vi "Parse JSON detailed err.vi"(8 "error in (no error)":errorcluster, 11 "JSON string in":string) -> (0 "error out":errorcluster, 3 "long err description out":string)   [LabVIEW 2018, in "LabView-0mq-Jl_Roundtrip_lib.lvlib"]
uses:
  LabView-0mq-Jl_Roundtrip_lib.lvlib
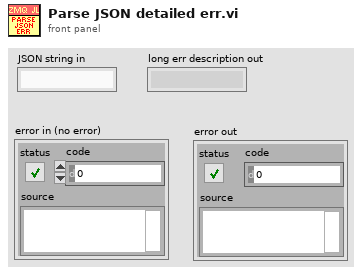
[diagram p1: front panel]
types:
  T1 = cluster{"status":bool, "code":i32, "source":string, "longdescr":string}
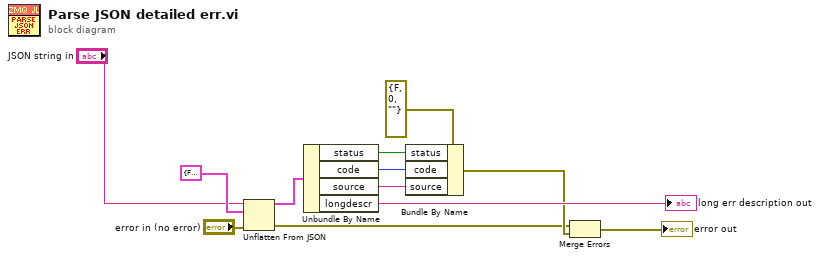
[diagram p0: block diagram]
diagram:
  n1 = Unflatten From JSON(JSON string="JSON string in", type and defaults=T1 {"status"=FALSE, "code"=0, "source"="", "longdescr"=""} ("error  with longdescr"), error in (no error)="error in (no error)") -> (value=w8:T1, error out=w4:errorcluster)  [unwired: 4 in]
  n2 = Unbundle By Name(w8) -> ("status"=w9:bool, "code"=w10:i32, "source"=w11:string, "longdescr"=→"long err description out":string)
  n3 = Bundle By Name(cluster=errorcluster {"status"=FALSE, "code"=0, "source"=""} ("error out 2"), "status"=w9, "code"=w10, "source"=w11) -> (w6:errorcluster)
  n4 = Merge Errors(w4, w6) -> (→"error out":errorcluster)
